vi "Signal Generator.vi"(8 "Ajuste Negativo (10 ^-4)":dbl, 9 "Ajuste Positivo (10 ^-4)":dbl, 11 "data":dbl=1.7 format="%#_13g") -> ()   [LabVIEW 2013]
uses:
  <vilib>/DAQmx/write.llb/DAQmx Write (Analog DBL 1Chan 1Samp).vi
panel:
  in  "OK Button":bool
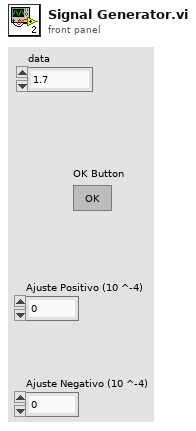
[diagram p1: front panel]
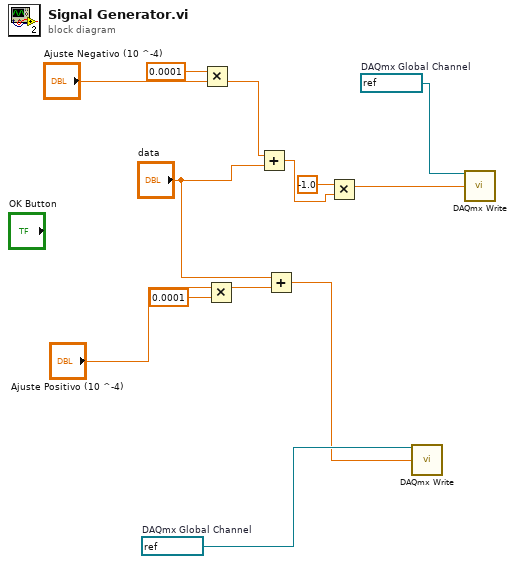
[diagram p0: block diagram]
diagram:
  w11 = refnum<k21> "Teste2"  # DAQmx Global Channel
  w10 = refnum<k21> "Teste1"  # DAQmx Global Channel
  n1 = Multiply(x=0.0001, y="Ajuste Negativo (10 ^-4)") -> (x*y=w2:dbl)
  n2 = Multiply(x="Ajuste Positivo (10 ^-4)", y=0.0001) -> (x*y=w4:dbl)
  n3 = Add(x=w2, y="data") -> (x+y=w5:dbl)
  n4 = Add(x="data", y=w4) -> (x+y=w9:dbl)
  n5 = Multiply(x=-1.0, y=w5) -> (x*y=w12:dbl)
  n6 = call-poly <vilib>:"DAQmx Write.vi"("task/channels in"=w10, "data"=w9) -> ()  [unwired: 11 in, 3 out]
  n7 = call-poly <vilib>:"DAQmx Write.vi"("task/channels in"=w11, "data"=w12) -> ()  [unwired: 11 in, 3 out]
